vi "String to int.vi"(11 "Int as Text":string) -> (3 "Int":i32)   [LabVIEW 2018, in "Receipt Parsing.lvlib"]
uses:
  Receipt Parsing.lvlib
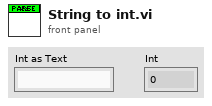
[diagram p1: front panel]
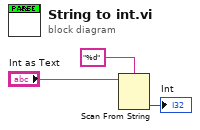
[diagram p0: block diagram]
diagram:
  n1 = Scan From String(format string="%d", input string="Int as Text") -> (output 1=→"Int":i32)  [unwired: 3 in, 3 out]
